vi "Error Handler.vi"(8 "error in (no error)":errorcluster, 11 "Dispatcher in":refnum<class "Dispatcher Thread.lvclass">) -> (0 "error out":errorcluster, 3 "Dispatcher out":refnum<class "Dispatcher Thread.lvclass">)   [LabVIEW 2017, in "DSF Core.lvlib" / "Dispatcher Thread.lvclass"]
uses:
  Dispatcher Thread.lvclass
  Dispatcher Thread.lvclass/Dispatcher Thread.ctl
  Interfaces/Interface/Interface.lvclass/Interface.ctl
  Interfaces/Interface/Write Error.vi
  Interfaces/Interface/Write Error Queue.vi
  Interfaces/Dispatcher/Dispatcher Interface.lvclass
  C:/Git/DSF/Data Sharing Framework/Source/Core/Engine/Classes/Interfaces/Interface/Interface.lvclass
  Interfaces/Dispatcher/Class Name.vi
  Interfaces/Interface/Errors.vi
  Interfaces/Dispatcher/Error Timeout.vi
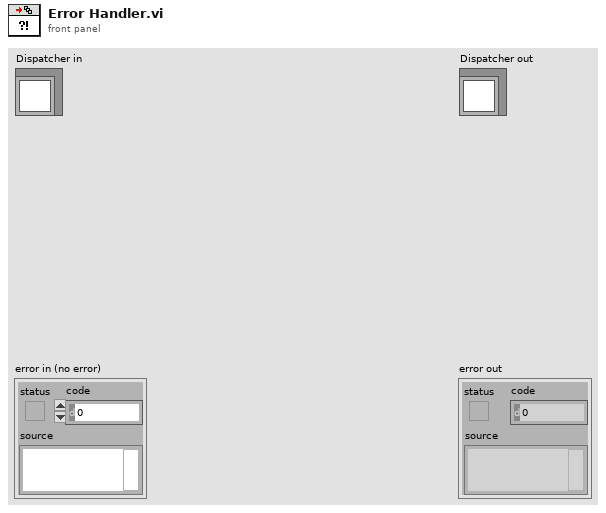
[diagram p1: front panel]
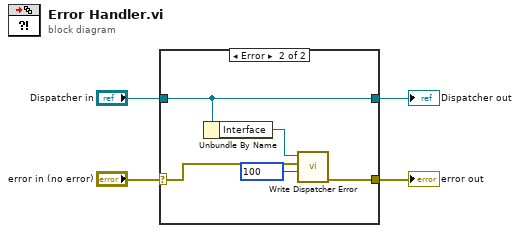
[diagram p0: block diagram]
diagram:
  n1 = case shown="Error" "error in (no error)" {
    selector: "error in (no error)" -> [w6 w8]
    tunnel: [w6 w11] -> w3
    tunnel: "Dispatcher in" -> [w5 w9]
    tunnel: [w5 w9] -> w1
    frame No Error {
    }
    frame Error {
      n2 = Unbundle By Name(w9) -> ("Interface"=w7:refnum<class "Dispatcher Interface.lvclass">)
      n3 = call "Write Dispatcher Error.vi"("timeout in ms (0)"=100, "error"=w8, "Dispatcher Interface in"=w7) -> ("error out"=w11:errorcluster)  [unwired: 7 in, 1 out]
    }
  }
  "error out" <- w3
  "Dispatcher out" <- w1
